vi "tracking+matching_gige_mit_2_pattern.vi"() -> ()   [LabVIEW 2014]
uses:
  <vilib>/userdefined/High Color/IMAQdx.ctl
  <vilib>/vision/Avi1.llb/AviRefnum.ctl
  <vilib>/vision/driver/NI_Vision_Acquisition_Software.lvlib
  <vilib>/vision/NI_Vision_Development_Module.lvlib
  <resource>/objmgr/imaqdx.rc
panel:
  in  "Aufnahme Starten":bool
  in  "Max Data Size":u32=10000
  out "Selected Path":path
  in  "Frames Per Second":u32=20
  in  "BayerPattern":u32(ring)=5 items=["None", "GB", "GR", "BG", "RG", "Use Hardware Value"]
  out "ValueString":string
  out "ValueBool":bool
  out "IPAddress":string
  in  "pattern2":bool
  in  "Pattern2 Farbe":u32(colorbox)=16711680
  in  "x":i32
  in  "y":i32
  out "Pattern1 2":T1(plugin-control)
  in  "Template File Path (Pattern Matching 2)":path=path "C:/Users/Kroll/Desktop/Test_04012016/Pattern/pattern_1412.png"
  out "date/time string":string
  in  "file path (dialog if empty)":path=path "I:/123.txt"
  in  "Länge der Spur":i32=50
  out "Pattern1":T1(plugin-control)
  in  "Template File Path (Pattern Matching 1)":path=path "C:/Users/Kroll/Desktop/Test_04012016/Pattern/pattern_1412.png"
  out "Image 2":T1(plugin-control)
  in  "Programm anhalten":bool
  in  "Parameters Pattern":T2={"Number of Matches Requested"=1, "Minimum Match Score"=800.0, "Angle Ranges"=[{"Start Angle"=-180.0, "End Angle"=180.0}, {"Start Angle"=0.0, "End Angle"=360.0}]}
  in  "Mittelpunktgröße":sgl
  in  "millisecond multiple":u32
  out "Processed Frames/s":dbl
  in  "Länge des Pfeils":sgl=80.0
  out "Acquired Frames/s":dbl
  in  "pattern1":bool
  in  "Pattern1 Farbe":u32(colorbox)=16711680
  in  "x":i32
  in  "y":i32
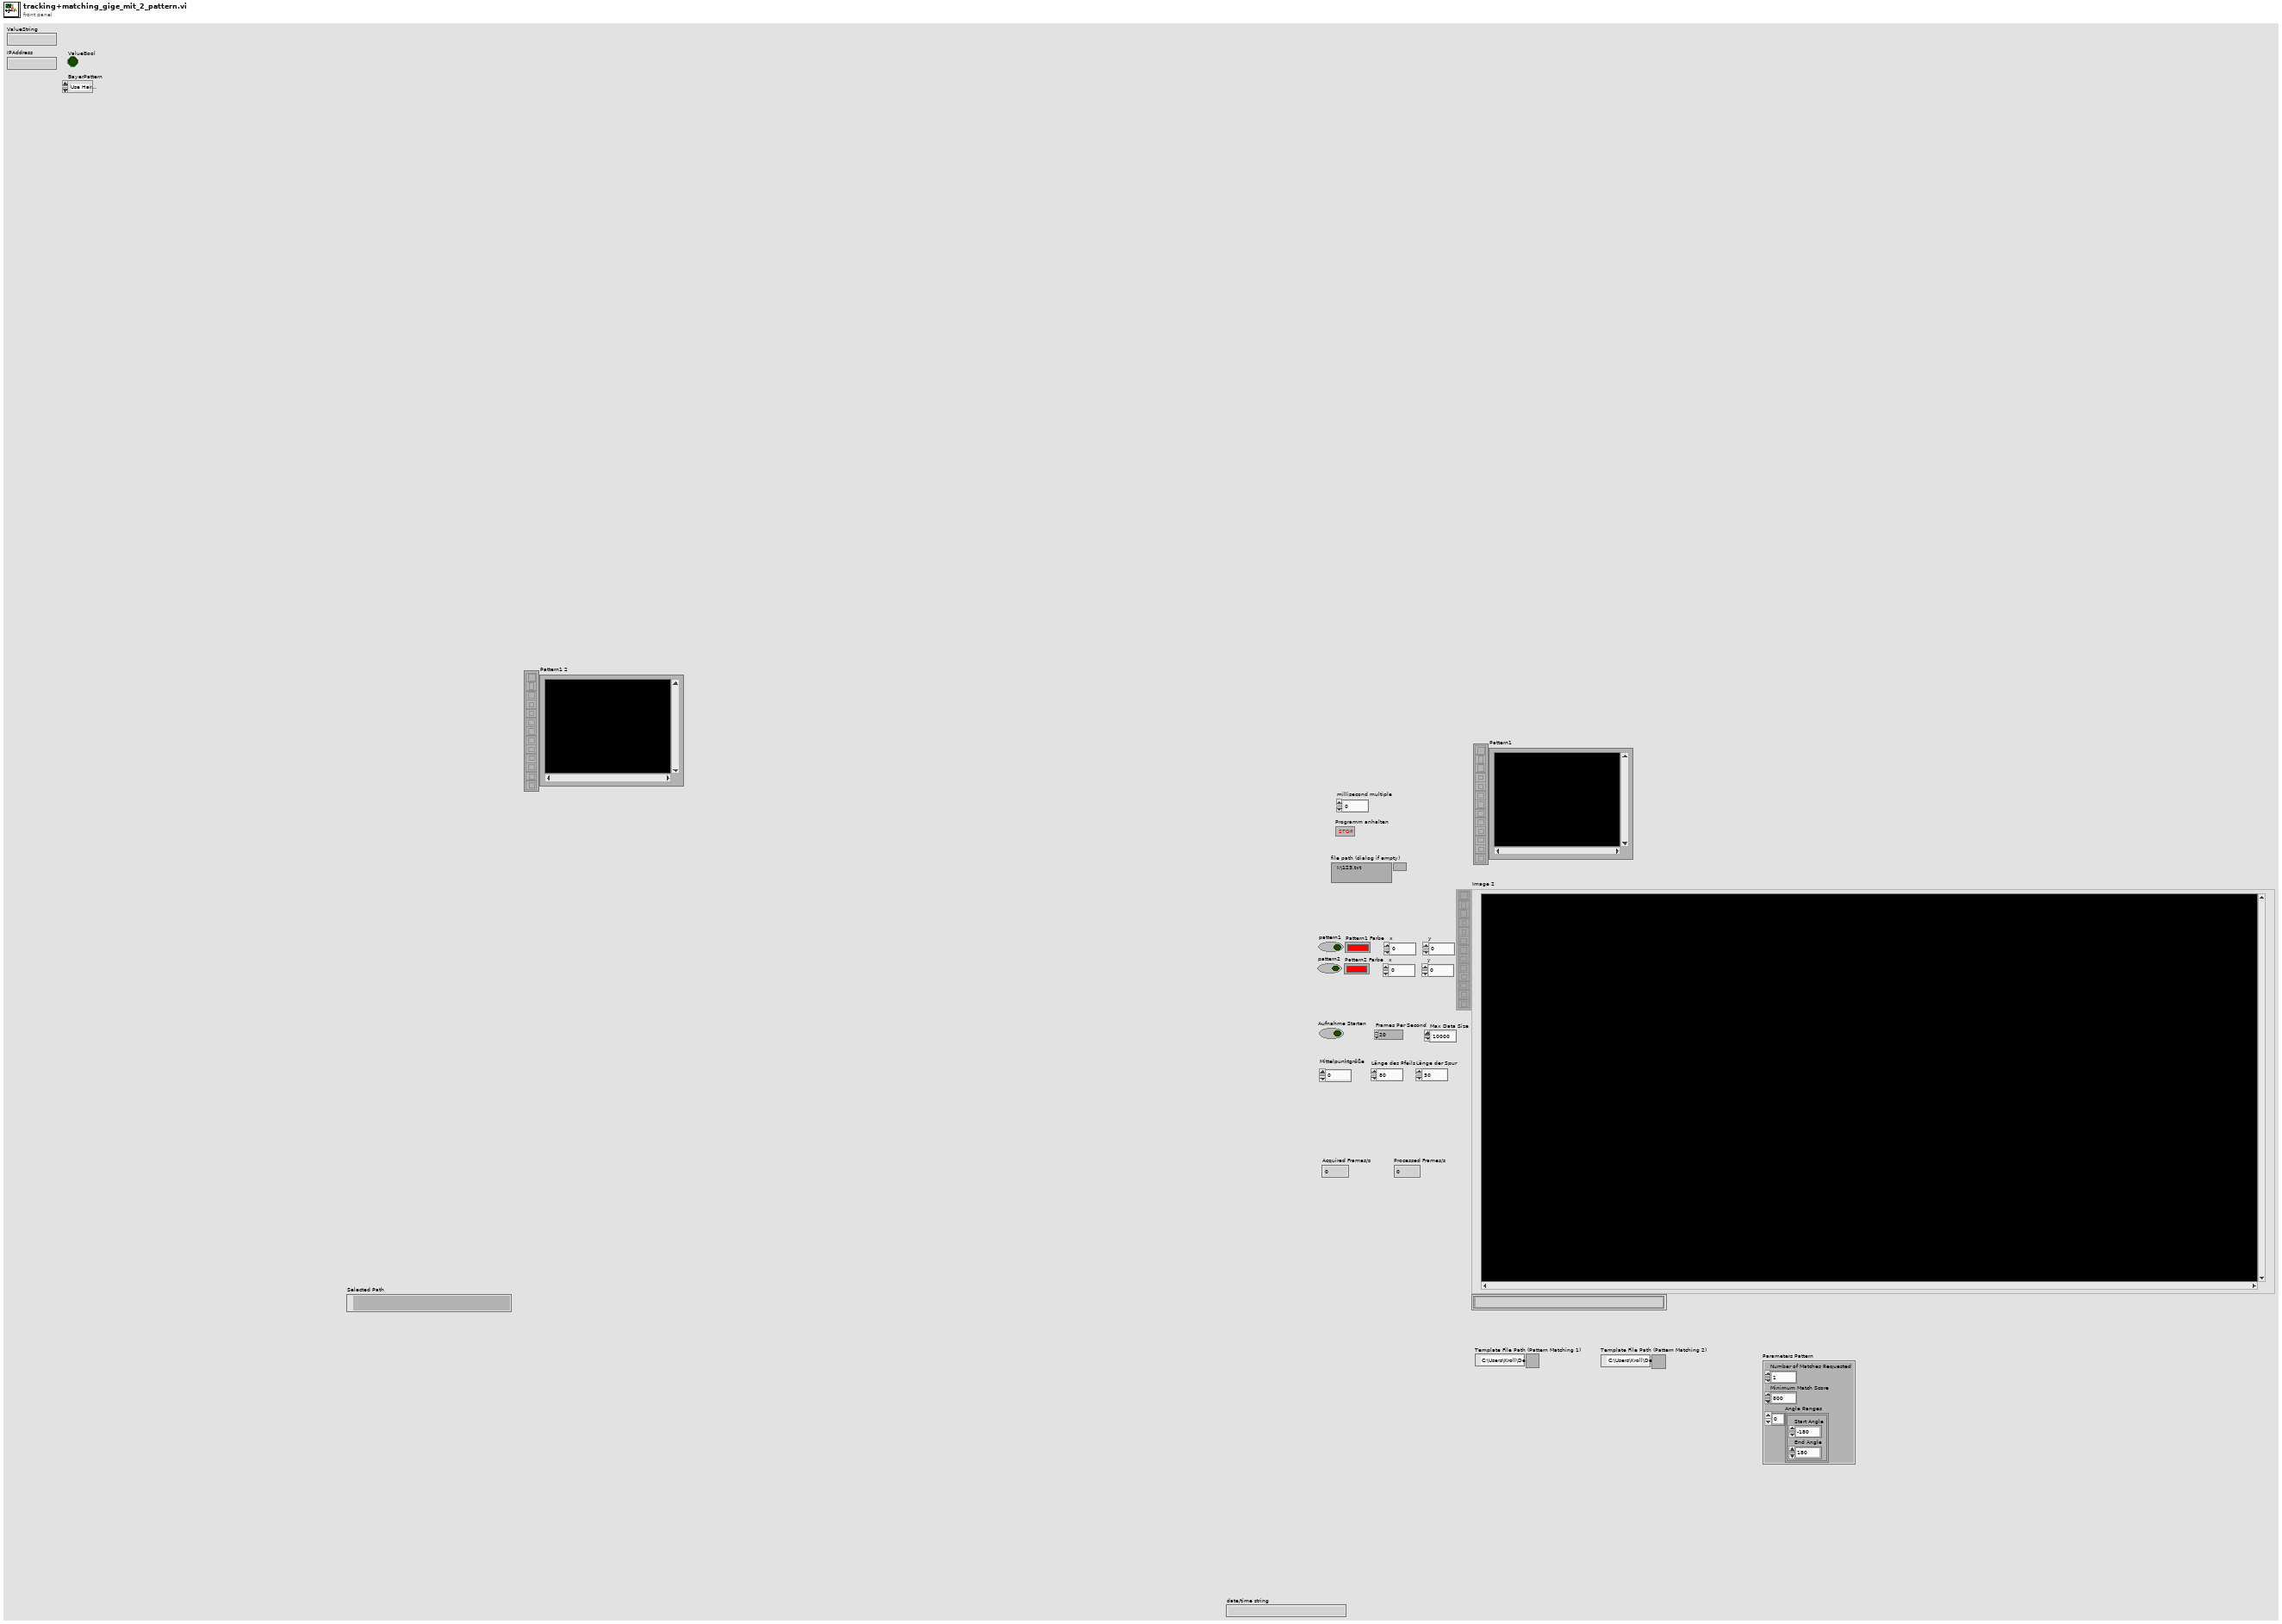
[diagram p1: front panel]
types:
  T1 = typedef "IMAQ Image.ctl" = refnum<image>
  T2 = cluster{"Number of Matches Requested":i32, "Minimum Match Score":sgl, "Angle Ranges":cluster{"Start Angle":sgl, "End Angle":sgl}[]}
  T3 = typedef "IMAQdx.ctl" = refnum<k21>
  T4 = cluster{"Number of Histogram Bins":i32, "Blending Parameter (%)":dbl, "Maximum Iterations":i32}
  T5 = typedef "Image Type" = u32
  T6 = enum16{"open", "replace", "create", "open or create", "replace or create", "replace or create with confirmation"}
  T7 = typedef "AviRefnum.ctl" = refnum<k1>
  T8 = enum32{"existing file", "new file", "new or existing file", "existing dir", "new dir", "new or existing dir", "existing file (use LLBs)", "new file (use LLBs)", "new or existing file (use LLBs)", "new or existing file or directory (use LLBs)"}
  T9 = typedef "IMAQ Object Tracking Session.ctl" = refnum<k20>
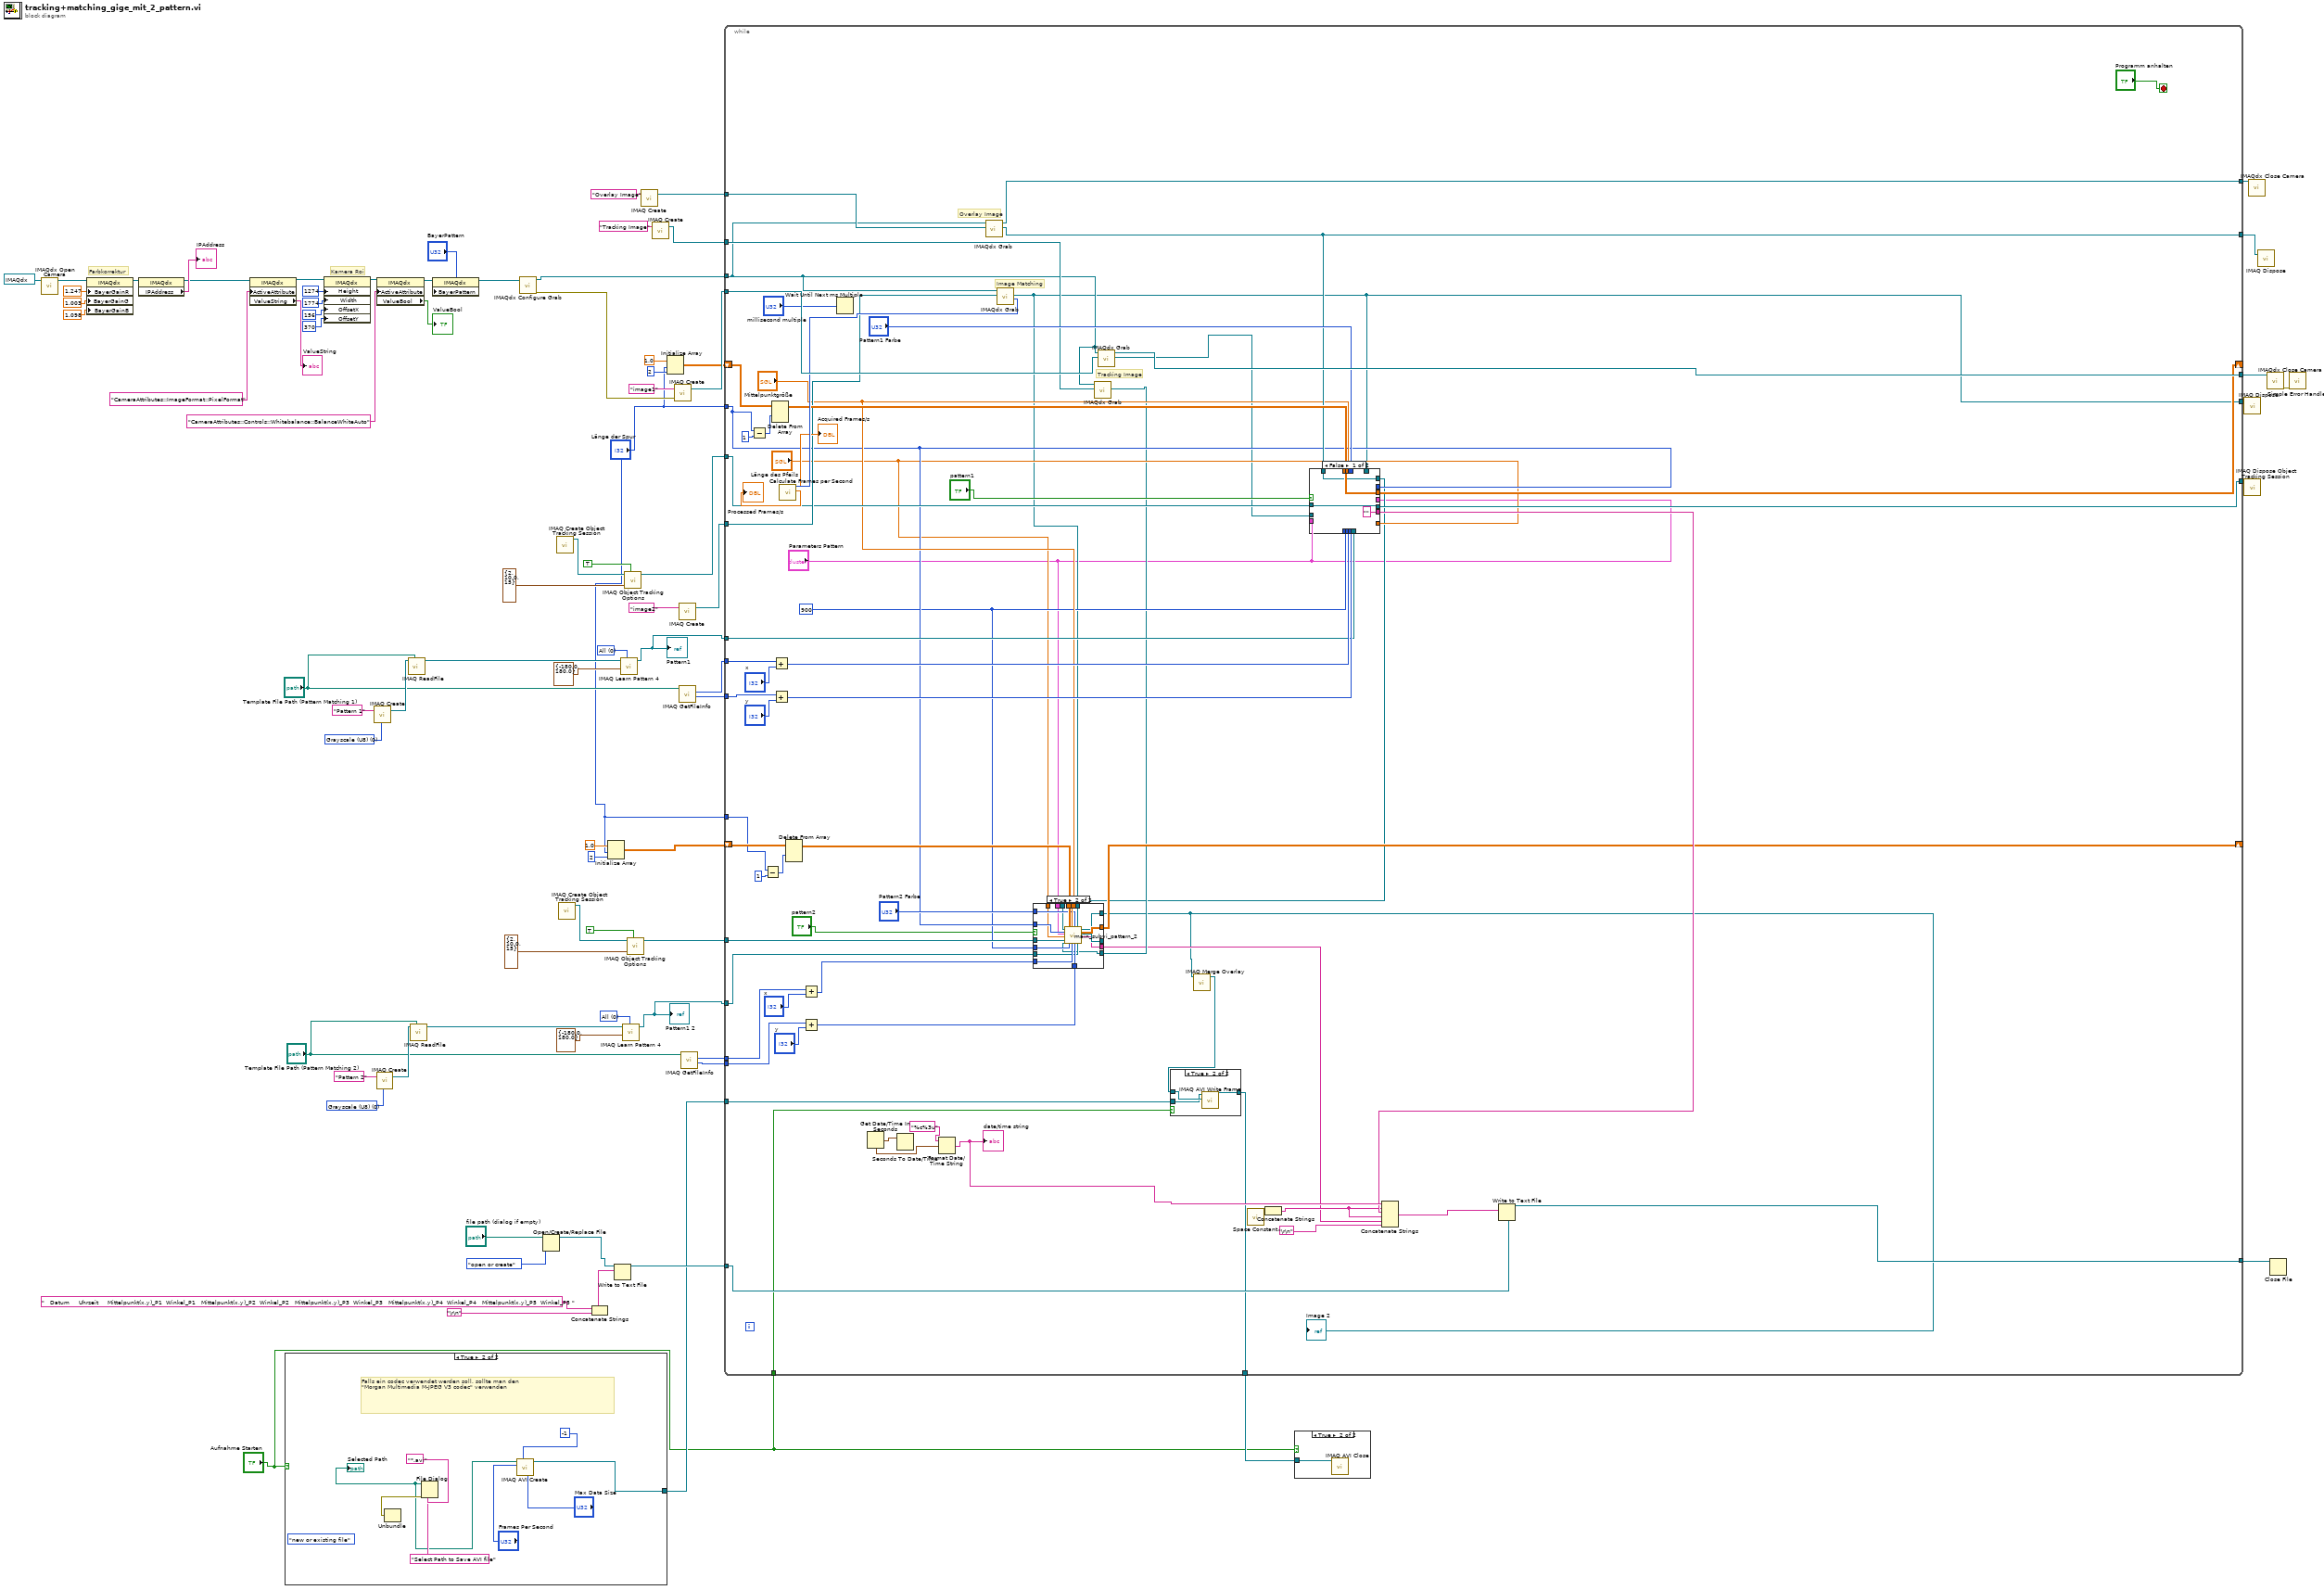
[diagram p0: block diagram]
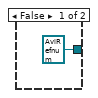
[diagram p3: hidden frame]
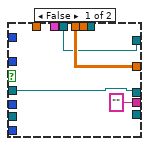
[diagram p5: hidden frame]
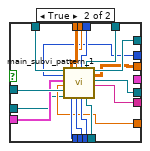
[diagram p6: hidden frame]
diagram:
  w40 = T5 0 items=["Grayscale (U8)", "Grayscale (I16)", "Grayscale (SGL)", "Complex (CSG)", "RGB (U32)", "HSL (U32)", "RGB (U64)", "Grayscale (U16)"] ("Image Type")
  w44 = 0 items=["All", "Low Discrepancy Sampling", "Grayscale Value Pyramid", "Gradients Pyramid"] ("Algorithm")
  w65 = T5 0 items=["Grayscale (U8)", "Grayscale (I16)", "Grayscale (SGL)", "Complex (CSG)", "RGB (U32)", "HSL (U32)", "RGB (U64)", "Grayscale (U16)"] ("Image Type")
  w69 = 0 items=["All", "Low Discrepancy Sampling", "Grayscale Value Pyramid", "Gradients Pyramid"] ("Algorithm")
  # "Kamera Roi"
  # "Farbkorrektur"
  n1 = call <vilib>:"IMAQdx Open Camera.vi"("Session In"=T3 "cam0") -> ("Session Out"=w13:T3)  [unwired: 9 in, 1 out]
  n2 = property class="IMAQdx"(reference=w13, "BayerGainR"=1.247, "BayerGainG"=1.003, "BayerGainB"=1.098) -> (reference out=w17:T3)  [unwired: 1 in, 1 out]
  n3 = property class="IMAQdx"(reference=w17) -> (reference out=w5:T3, "IPAddress"=→"IPAddress":string)  [unwired: 1 in, 1 out]
  n4 = property class="IMAQdx"(reference=w5, "ActiveAttribute"="CameraAttributes::ImageFormat::PixelFormat") -> (reference out=w10:T3, "ValueString"=→"ValueString":string)  [unwired: 1 in, 1 out]
  n5 = case shown="True" "Aufnahme Starten" {
    tunnel: [T7 refnum ("Avi Refnum") w86] -> w3
    frame False {
    }
    frame True {
      (unwired) T8."new or existing file" ("select mode (2)")
      # "Falls ein codec verwendet werden soll, sollte man den \n\"Morgan Multimedia M-JPEG V3 codec\" verwenden"
      n6 = File Dialog(6:"*.avi" ("pattern"), 7:"Select Path to Save AVI file" ("prompt")) -> (0:w89:errorcluster, 3:w88:path)  [unwired: 1 in, 6 out]
      "Selected Path" <- w88
      n7 = Unbundle(w89) -> ()  [unwired: 3 out]
      n8 = call "IMAQ AVI Create"("Max Data Size"="Max Data Size", "quality"=-1, "Frames Per Second"="Frames Per Second", "AVI Path"=w88) -> ("Avi Refnum"=w86:T7)  [unwired: 6 in, 1 out]
    }
  }
  n9 = property class="IMAQdx"(reference=w10, "Height"=u32 1274, "Width"=u32 1774, "OffsetX"=u32 156, "OffsetY"=u32 370) -> (reference out=w11:T3)  [unwired: 1 in, 1 out]
  n10 = call "IMAQ Create"("Image Name"="Pattern 1", "Image Type"=w65) -> ("New Image"=w66:T1)  [unwired: 3 in, 1 out]
  n11 = call "IMAQ Create"("Image Name"="Pattern 2", "Image Type"=w40) -> ("New Image"=w41:T1)  [unwired: 3 in, 1 out]
  n12 = property class="IMAQdx"(reference=w11, "ActiveAttribute"="CameraAttributes::Controls::Whitebalance::BalanceWhiteAuto") -> (reference out=w21:T3, "ValueBool"=→"ValueBool":bool)  [unwired: 1 in, 1 out]
  n13 = call "IMAQ ReadFile"("File Path"="Template File Path (Pattern Matching 1)", "Image"=w66) -> ("Image Out"=w62:T1)  [unwired: 5 in, 4 out]
  n14 = call "IMAQ ReadFile"("File Path"="Template File Path (Pattern Matching 2)", "Image"=w41) -> ("Image Out"=w38:T1)  [unwired: 5 in, 4 out]
  n15 = property class="IMAQdx"(reference=w21, "BayerPattern"="BayerPattern") -> (reference out=w4:T3)  [unwired: 1 in, 1 out]
  n16 = call <vilib>:"IMAQdx Configure Grab.vi"("Session In"=w4) -> ("error out"=w83:errorcluster, "Session Out"=w81:T3)  [unwired: 9 in]
  n17 = Open/Create/Replace File(file path (use dialog)="file path (dialog if empty)", operation (0:open)=T6."open or create") -> (refnum out=w51:refnum<file>)  [unwired: 4 in, 2 out]
  n18 = call "IMAQ Create Object Tracking Session"() -> ("Object Tracking Session"=w61:T9)  [unwired: 1 in, 10 out]
  n19 = call "IMAQ Create Object Tracking Session"() -> ("Object Tracking Session"=w37:T9)  [unwired: 1 in, 10 out]
  n20 = Concatenate Strings("   Datum     Uhrzeit     Mittelpunkt(x,y)_P1  Winkel_P1   Mittelpunkt(x,y)_P2  Winkel_P2   Mittelpunkt(x,y)_P3  Winkel_P3   Mittelpunkt(x,y)_P4  Winkel_P4   Mittelpunkt(x,y)_P5  Winkel_P5 " ("string"), "\r\n") -> (w49:string)
  n21 = Initialize Array "Initialize Array"(1.0 ("element"), "Länge der Spur", 2 ("dimension size")) -> (w28:dbl[][])
  n22 = Write to Text File(file (use dialog)=w51, text=w49) -> (refnum out=w47:refnum<file>)  [unwired: 2 in, 2 out]
  n23 = call "IMAQ Learn Pattern 4"("Algorithm"=w69, "Angle Range"=cluster{"Start Angle":sgl, "End Angle":sgl} {"Start Angle"=-180.0, "End Angle"=180.0}, "Image"=w62) -> ("Template Image Out"=w63:T1)  [unwired: 6 in, 2 out]
  "Pattern1" <- w63
  n24 = call "IMAQ Learn Pattern 4"("Algorithm"=w44, "Angle Range"=cluster{"Start Angle":sgl, "End Angle":sgl} {"Start Angle"=-180.0, "End Angle"=180.0}, "Image"=w38) -> ("Template Image Out"=w33:T1)  [unwired: 6 in, 2 out]
  "Pattern1 2" <- w33
  n25 = call-poly "IMAQ Object Tracking Options"("Get/Set (Get)"=TRUE, "Mean Shift Options in"=T4 {"Number of Histogram Bins"=2, "Blending Parameter (%)"=10.0, "Maximum Iterations"=15}, "Object Tracking Session In"=w61) -> ("Object Tracking Session Out"=w60:T9)  [unwired: 6 in, 2 out]
  n26 = call-poly "IMAQ Object Tracking Options"("Get/Set (Get)"=TRUE, "Mean Shift Options in"=T4 {"Number of Histogram Bins"=2, "Blending Parameter (%)"=10.0, "Maximum Iterations"=15}, "Object Tracking Session In"=w37) -> ("Object Tracking Session Out"=w34:T9)  [unwired: 6 in, 2 out]
  n27 = call "IMAQ Create"("Image Name"="Overlay Image") -> ("New Image"=w57:T1)  [unwired: 4 in, 1 out]
  n28 = call "IMAQ Create"("Image Name"="Tracking Image") -> ("New Image"=w25:T1)  [unwired: 4 in, 1 out]
  n29 = Initialize Array "Initialize Array"(1.0 ("element"), "Länge der Spur", 2 ("dimension size")) -> (w71:dbl[][])
  n30 = call "IMAQ Create"("Image Name"="image1", "error in (no error)"=w83) -> ("New Image"=w80:T1)  [unwired: 3 in, 1 out]
  n31 = call "IMAQ Create"("Image Name"="image2") -> ("New Image"=w76:T1)  [unwired: 4 in, 1 out]
  n32 = call "IMAQ GetFileInfo"("File Path"="Template File Path (Pattern Matching 1)") -> ("Y Resolution"=w73:i32, "X Resolution"=w74:i32)  [unwired: 4 in, 5 out]
  n33 = call "IMAQ GetFileInfo"("File Path"="Template File Path (Pattern Matching 2)") -> ("Y Resolution"=w31:i32, "X Resolution"=w32:i32)  [unwired: 4 in, 5 out]
  n34 = while {
    tunnel: w81 -> [w105]
    tunnel: w80 -> [w161]
    tunnel: [w162] -> w78
    tunnel: [w102] -> w75
    tunnel: w76 -> [w147]
    tunnel: w74 -> [w148]
    tunnel: w73 -> [w149]
    shift-right: [w140] -> _
    shift-left: w71 -> [w156]
    tunnel: "Länge der Spur" -> [w117]
    tunnel: w63 -> [w137]
    tunnel: w60 -> [w141]
    tunnel: [w146] -> w58
    tunnel: w57 -> [w143]
    tunnel: [w138] -> w56
    tunnel: [w142] -> w55
    tunnel: w47 -> [w134]
    tunnel: [w130] -> w46
    tunnel: w34 -> [w116]
    tunnel: w33 -> [w112]
    tunnel: w32 -> [w127]
    tunnel: w31 -> [w126]
    shift-right: [w120] -> _
    shift-left: w28 -> [w123]
    tunnel: "Länge der Spur" -> [w122]
    tunnel: w25 -> [w106]
    tunnel: w3 -> [w97]
    tunnel: [w96] -> w2
    tunnel: "Aufnahme Starten" -> [w95]
    stop <- "Programm anhalten" stop-if-true
    w115 = 900 ("Minimum Score")
    # "Overlay Image"
    # "Image Matching"
    # "Tracking Image"
    n35 = Subtract(x=w117, y=1) -> (x-y=w153:i32)
    n36 = Subtract(x=w122, y=1) -> (x-y=w124:i32)
    n37 = Delete From Array "Delete From Array"(array=w156, index (row)=w153) -> (array with subset deleted=w155:dbl[][])  [unwired: 2 in, 1 out]
    n38 = Add(x=w148, y="x") -> (x+y=w145:i32)
    n39 = Add(x=w149, y="y") -> (x+y=w144:i32)
    n40 = Delete From Array "Delete From Array"(array=w123, index (row)=w124) -> (array with subset deleted=w121:dbl[][])  [unwired: 2 in, 1 out]
    n41 = Add(x=w127, y="x") -> (x+y=w113:i32)
    n42 = Add(x=w126, y="y") -> (x+y=w114:i32)
    n43 = Wait Until Next ms Multiple(millisecond multiple="millisecond multiple") -> ()  [unwired: 1 out]
    n44 = Get Date/Time In Seconds() -> (seconds since 1Jan1904=w133:timestamp)
    n45 = Seconds To Date/Time(time stamp (now)=w133) -> ()  [unwired: 1 in, 1 out]
    n46 = Format Date/Time String(time format string (%c)="%c%3u", seconds (now)=w133) -> (date/time string=w131:string)  [unwired: 1 in]
    "date/time string" <- w131
    n47 = call <vilib>:"IMAQdx Grab.vi"("Image In"=w143, "Session In"=w105) -> ("Image Out"=w138:T1, "Session Out"=w142:T3)  [unwired: 6 in, 2 out]
    n48 = call <vilib>:"IMAQdx Grab.vi"("Image In"=w147, "Session In"=w105) -> ("Buffer Number Out"=w159:u32, "Image Out"=w102:T1)  [unwired: 6 in, 2 out]
    n49 = call <vilib>:"Calculate Frames per Second.vi"("Buffer Number"=w159) -> ("Processed Frames/s"=→"Processed Frames/s":dbl, "Acquired Frames/s"=→"Acquired Frames/s":dbl)  [unwired: 8 in, 1 out]
    n50 = call <vilib>:"IMAQdx Grab.vi"("Image In"=w106, "Session In"=w105) -> ("Image Out"=w104:T1)  [unwired: 6 in, 3 out]
    n51 = call <vilib>:"IMAQdx Grab.vi"("Image In"=w161, "Session In"=w105) -> ("Image Out"=w110:T1, "Session Out"=w162:T3)  [unwired: 6 in, 2 out]
    n52 = call <vilib>:"Space Constant.vi"() -> ("String"=w136:string)
    n53 = Concatenate Strings(w136, w136) -> (w100:string)
    n54 = case shown="False" "pattern1" {
      tunnel: w155 -> [w191 w201]
      tunnel: "Länge des Pfeils" -> [_ w196]
      tunnel: "Mittelpunktgröße" -> [_ w200]
      tunnel: w115 -> [_ w203]
      tunnel: [w192 w208] -> w146
      tunnel: w145 -> [_ w204]
      tunnel: w144 -> [_ w205]
      tunnel: w102 -> [_ w199]
      tunnel: w141 -> [w192 w202]
      tunnel: w117 -> [_ w193]
      tunnel: [w191 w209] -> w140
      tunnel: "Pattern1 Farbe" -> [_ w194]
      tunnel: w138 -> [w189 w198]
      tunnel: w137 -> [_ w206]
      tunnel: ["" ("String") w207] -> w129
      tunnel: "Parameters Pattern" -> [_ _]
      tunnel: [w189 w210] -> w103
      tunnel: w110 -> [_ w195]
      tunnel: "Parameters Pattern" -> [_ w197]
      frame False {
      }
      frame True {
        n55 = call "main_subvi_pattern_1.vi"("Refnum Original Bild"=w198, "Länge der Spur"=w193, "Parameters Pattern"=w197, "Länge des Pfeils"=w196, "Object Tracking Session Out in"=w202, "Refnum Tracking"=w195, "Array in"=w201, "Minimum Score"=w203, "Mittelpunktgröße"=w200, "Numeric 2"=w204, "Pattern1 Farbe"=w194, "Numeric"=w205, "Image Matching"=w199, "Template Image In"=w206) -> ("Refnum OUt"=w210:T1, "Array out"=w209:dbl[][], "Object Tracking Session Out out"=w208:T9, "String"=w207:string)  [unwired: 2 in]
      }
    }
    n56 = case shown="True" "pattern2" {
      tunnel: [w168 w188] -> _
      tunnel: [w169 w187] -> w120
      tunnel: ["" ("String") w186] -> w98
      tunnel: [w167 w185] -> w93
      tunnel: w121 -> [w169 w184]
      tunnel: w102 -> [_ w183]
      tunnel: "Mittelpunktgröße" -> [_ w182]
      tunnel: "Pattern2 Farbe" -> [_ w181]
      tunnel: w117 -> [_ w180]
      tunnel: w116 -> [w168 w179]
      tunnel: w103 -> [w167 w178]
      tunnel: "Parameters Pattern" -> [_ w177]
      tunnel: w115 -> [_ w176]
      tunnel: w114 -> [_ w175]
      tunnel: w113 -> [_ w174]
      tunnel: w112 -> [_ w173]
      tunnel: "Länge des Pfeils" -> [_ w172]
      tunnel: w104 -> [_ w171]
      frame False {
      }
      frame True {
        n57 = call "main_subvi_pattern_2.vi"("Refnum Original Bild"=w178, "Länge der Spur"=w180, "Parameters Pattern"=w177, "Länge des Pfeils"=w172, "Object Tracking Session Out in"=w179, "Refnum Tracking"=w171, "Array in"=w184, "Minimum Score"=w176, "Mittelpunktgröße"=w182, "Numeric 2"=w174, "Pattern1 Farbe"=w181, "Numeric"=w175, "Image Matching"=w183, "Template Image In"=w173) -> ("Refnum OUt"=w185:T1, "Array out"=w187:dbl[][], "Object Tracking Session Out out"=w188:T9, "String"=w186:string)  [unwired: 2 in]
      }
    }
    "Image 2" <- w93
    n58 = call "IMAQ Merge Overlay"("Image Src"=w93) -> ("Image Dst Out"=w94:T1)  [unwired: 9 in, 1 out]
    n59 = case shown="True" w95 {
      tunnel: w94 -> [_ w166]
      tunnel: [w163 w165] -> w96
      tunnel: w97 -> [w163 w164]
      frame False {
      }
      frame True {
        n60 = call "IMAQ AVI Write Frame"("Image"=w166, "Avi Refnum"=w164) -> ("Avi Refnum (duplicate)"=w165:T7)  [unwired: 8 in, 1 out]
      }
    }
    n61 = Concatenate Strings(w131, w100, w129, w100, w98, "\r\n") -> (w135:string)
    n62 = Write to Text File(file (use dialog)=w134, text=w135) -> (refnum out=w130:refnum<file>)  [unwired: 2 in, 2 out]
  }
  n63 = case shown="True" "Aufnahme Starten" {
    tunnel: w2 -> [_ w211]
    frame False {
    }
    frame True {
      n64 = call "IMAQ AVI Close"("Avi Refnum"=w211) -> ()  [unwired: 10 in, 1 out]
    }
  }
  n65 = call "IMAQ Dispose"("Image"=w75) -> ()  [unwired: 5 in, 1 out]
  n66 = call "IMAQ Dispose Object Tracking Session"("Object Tracking Session"=w58) -> ()  [unwired: 1 in, 10 out]
  n67 = call <vilib>:"IMAQdx Close Camera.vi"("Session In"=w55) -> ()  [unwired: 10 in, 1 out]
  n68 = call "IMAQ Dispose"("Image"=w56) -> ()  [unwired: 5 in, 1 out]
  n69 = call <vilib>:"IMAQdx Close Camera.vi"("Session In"=w78) -> ("error out"=w79:errorcluster)  [unwired: 10 in]
  n70 = Close File(refnum=w46) -> ()  [unwired: 1 in, 2 out]
  n71 = call <vilib>:"Simple Error Handler.vi"("error in (no error)"=w79) -> ()  [unwired: 4 in, 5 out]
